vi "select_product (SubVI).vi"(11 "Item Selection":T1) -> (2 "Boolean":bool, 3 "Numeric":u16)   [LabVIEW 2020]
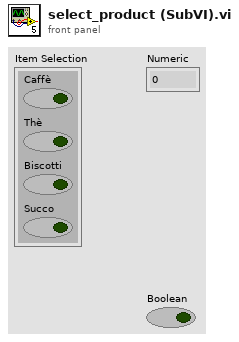
[diagram p1: front panel]
types:
  T1 = cluster{"Caffè":bool, "Thè":bool, "Biscotti":bool, "Succo":bool}
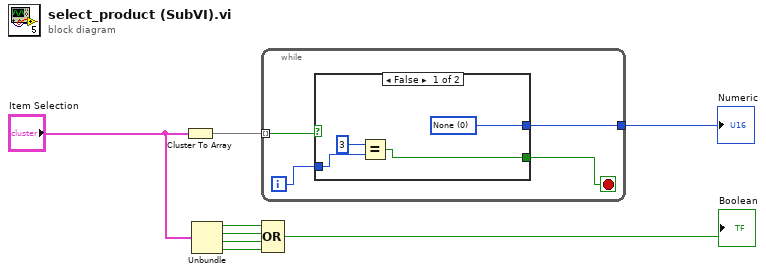
[diagram p0: block diagram]
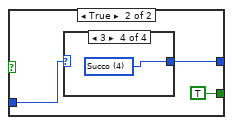
[diagram p2: hidden frame]
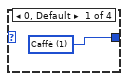
[diagram p3: hidden frame]
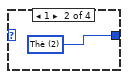
[diagram p4: hidden frame]
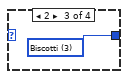
[diagram p5: hidden frame]
diagram:
  n1 = Cluster To Array(cluster="Item Selection") -> (array=w1:bool[])
  n2 = Unbundle("Item Selection") -> ("Caffè"=w4:bool, "Thè"=w5:bool, "Biscotti"=w6:bool, "Succo"=w7:bool)
  n3 = while {
    tunnel: [w12] -> w2
    tunnel: w1 -> [w11] mode=indexing
    i -> [w10]
    stop <- w9 stop-if-true
    n4 = case shown="False" w11 {
      tunnel: [w16 w19] -> w12
      tunnel: w10 -> [w14 w18]
      tunnel: [w15 TRUE] -> w9
      frame False {
        w16 = u16 0 items=["None", "Caffè", "Thè", "Biscotti", "Succo"]
        n5 = Equal?(x=3, y=w14) -> (x = y?=w15:bool)
      }
      frame True {
        n6 = case shown="3" w18 {
          tunnel: [w20 w21 w22 w23] -> w19
          frame 0, Default {
            w20 = u16 1 items=["None", "Caffè", "Thè", "Biscotti", "Succo"]
          }
          frame 1 {
            w21 = u16 2 items=["None", "Caffè", "Thè", "Biscotti", "Succo"]
          }
          frame 2 {
            w22 = u16 3 items=["None", "Caffè", "Thè", "Biscotti", "Succo"]
          }
          frame 3 {
            w23 = u16 4 items=["None", "Caffè", "Thè", "Biscotti", "Succo"]
          }
        }
      }
    }
  }
  "Numeric" <- w2
  n7 = Compound Arithmetic op=OR(w4, w5, w6, w7) -> (→"Boolean":bool)
